vi "Get_Coil_Traces.vi"() -> ()   [LabVIEW 2010]
panel:
  in  "path":path
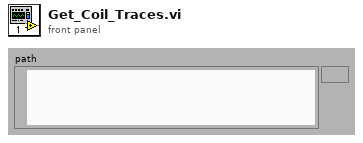
[diagram p1: front panel]
types:
  T1 = enum32{"existing file", "new file", "new or existing file", "existing dir", "new dir", "new or existing dir", "existing file (use LLBs)", "new file (use LLBs)", "new or existing file (use LLBs)", "new or existing file or directory (use LLBs)"}
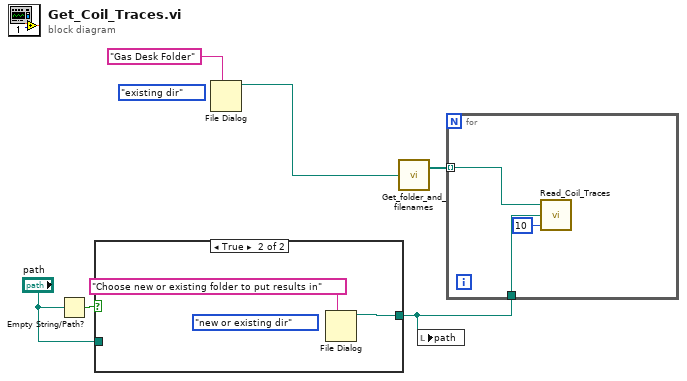
[diagram p0: block diagram]
diagram:
  (unwired) T1."existing dir" ("select mode (2)")
  n1 = Empty String/Path?(string/path="path") -> (empty?=w3:bool)
  n2 = case shown="True" w3 {
    tunnel: [w7 w8] -> w1
    tunnel: "path" -> [w7 _]
    frame False {
    }
    frame True {
      (unwired) T1."new or existing dir" ("select mode (2)")
      n3 = File Dialog(7:"Choose new or existing folder to put results in" ("prompt")) -> (3:w8:path)  [unwired: 6 in, 3 out]
    }
  }
  n4 = File Dialog(7:"Gas Desk Folder" ("prompt")) -> (3:w5:path)  [unwired: 6 in, 3 out]
  n5 = call "Get_folder_and_filenames.vi"("file path (dialog if empty)"=w5) -> ("Folders"=w4:path[])  [unwired: 1 out]
  n6 = local write "path"(w1) -> ()
  n7 = for {
    tunnel: w1 -> [w12]
    tunnel: w4 -> [w10] mode=indexing
    n8 = call "Read_Coil_Traces.vi"("Reduction"=10, "New Folder"=w12, "Gas Desk Folder"=w10) -> ()  [unwired: 1 in]
  }
